vi "源强与基线.vi"(5 "通量名称":string[](array[string]) caption="通量名称：", 6 "执行:调用时显示前面板":bool, 9 "通量in":dbl[](array[numeric])) -> (0 "源与基线灯":bool, 1 "源强out":dbl[](array[numeric]), 3 "通量out":dbl[](array[numeric]))   [LabVIEW 2020]
panel:
  in  "本底减除":dbl[](array[numeric]) caption="本底减除："
  in  "通道源强":dbl[](array[numeric]) caption="通道源强："
  out "面板开":bool
  in  "源与本底开关：":bool
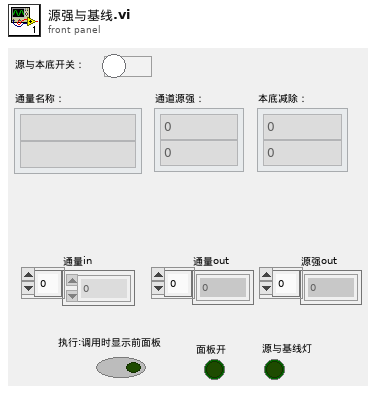
[diagram p1: front panel]
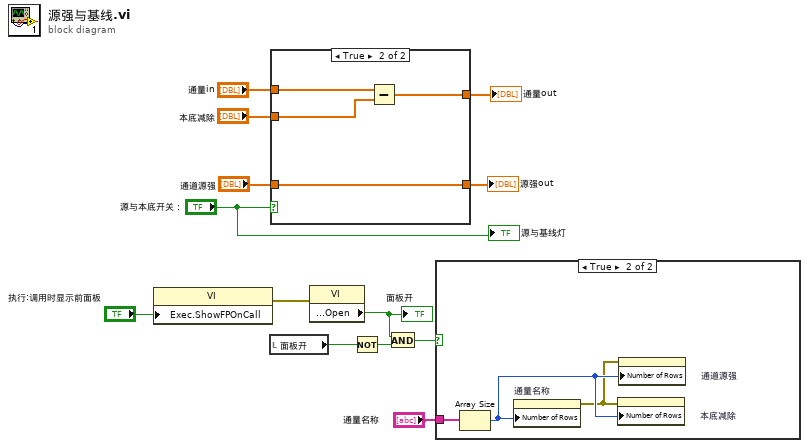
[diagram p0: block diagram]
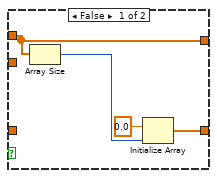
[diagram p3: hidden frame]
diagram:
  n1 = property class="VI"("Exec.ShowFPOnCall"="执行:调用时显示前面板") -> (error out=w11:errorcluster)  [unwired: 2 in, 1 out]
  n2 = local read "面板开"() -> (w10:bool)
  n3 = case shown="True" "源与本底开关：" {
    tunnel: "通量in" -> [w15 w20]
    tunnel: [w15 w19] -> w1
    tunnel: "通道源强" -> [_ w21]
    tunnel: "本底减除" -> [_ w18]
    tunnel: [w16 w21] -> w4
    frame False {
      n4 = Array Size(array=w15) -> (size(s)=w14:i32)
      n5 = Initialize Array(0.0 ("元素"), w14) -> (w16:dbl[])
    }
    frame True {
      n6 = Subtract(x=w20, y=w18) -> (x-y=w19:dbl[])
    }
  }
  "通量out" <- w1
  "源强out" <- w4
  n7 = property class="VI"(error in=w11) -> ("Front Panel.Open"=w8:bool)  [unwired: 1 in, 2 out]
  "面板开" <- w8
  n8 = Not(x=w10) -> (.not. x?=w9:bool)
  n9 = And(x=w8, y=w9) -> (x .and. y?=w7:bool)
  n10 = case shown="True" w7 {
    tunnel: "通量名称" -> [_ w24]
    frame False {
    }
    frame True {
      n11 = Array Size(array=w24) -> (size(s)=w23:i32)
      n12 = property on="通量名称" class="Arr (strict)"("Number of Rows"=w23) -> (error out=w22:errorcluster)  [unwired: 2 in, 1 out]
      n13 = property on="本底减除" class="Arr (strict)"(error in=w22, "Number of Rows"=w23) -> ()  [unwired: 1 in, 2 out]
      n14 = property on="通道源强" class="Arr (strict)"(error in=w22, "Number of Rows"=w23) -> ()  [unwired: 1 in, 2 out]
    }
  }
  "源与基线灯" <- "源与本底开关："
